vi "Vector2DAngle.vi"(10 "Vector2D":T1) -> (2 "Angle":dbl)   [LabVIEW 2018]
uses:
  Vector2D.ctl
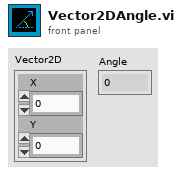
[diagram p1: front panel]
types:
  T1 = typedef "Vector2D.ctl" = cluster{"X":dbl, "Y":dbl}
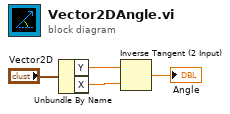
[diagram p0: block diagram]
diagram:
  n1 = Unbundle By Name("Vector2D") -> ("Y"=w3:dbl, "X"=w2:dbl)
  n2 = Inverse Tangent (2 Input)(1:w2, 2:w3) -> (0:→"Angle":dbl)
